vi "teampNight.vi"() -> ()   [LabVIEW 2010]
panel:
  in  "Temp Stop":dbl
  in  "Temp Step":dbl
  in  "Temp Start":dbl
  out "error out":errorcluster
  in  "error in (no error)":errorcluster
  in  "Step":dbl
  in  "Stop":dbl
  in  "Start":dbl
  in  "Path":path
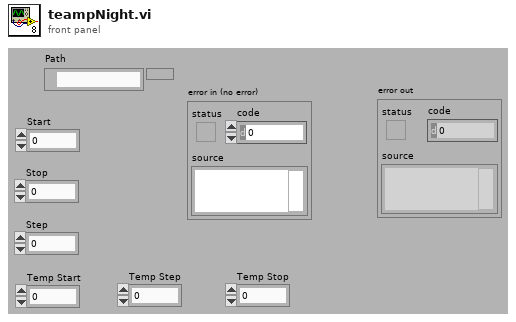
[diagram p1: front panel]
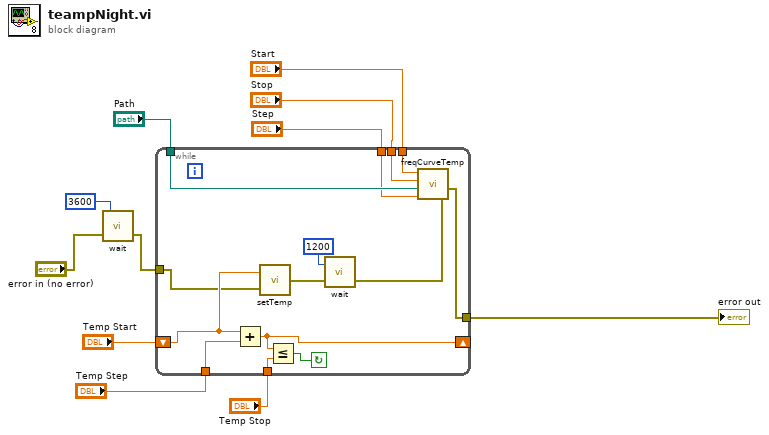
[diagram p0: block diagram]
diagram:
  n1 = call "wait.vi"("error in"="error in (no error)", "Wartezeit in Sek"=3600) -> ("error out"=w1:errorcluster)  [unwired: 1 in]
  n2 = while {
    tunnel: "Path" -> [w25]
    tunnel: w1 -> [w15]
    tunnel: [w24] -> w10
    tunnel: "Start" -> [w22]
    tunnel: "Stop" -> [w21]
    tunnel: "Step" -> [w20]
    shift-right: [w17] -> _
    shift-left: "Temp Start" -> [w16]
    tunnel: "Temp Step" -> [w18]
    tunnel: "Temp Stop" -> [w12]
    stop <- w19 continue-if-true
    n3 = Add(x=w16, y=w18) -> (x+y=w17:dbl)
    n4 = call "setTemp.vi"("error in (no error)"=w15, "Heizspannung"=w16) -> ("error out"=w14:errorcluster)
    n5 = Less Or Equal?(x=w17, y=w12) -> (x <= y?=w19:bool)
    n6 = call "wait.vi"("error in"=w14, "Wartezeit in Sek"=1200) -> ("error out"=w13:errorcluster)  [unwired: 1 in]
    n7 = call "freqCurveTemp.vi"("error in (no error)"=w13, "Step"=w20, "Path"=w25, "End"=w21, "Start"=w22) -> ("error out"=w24:errorcluster)  [unwired: 2 in]
  }
  "error out" <- w10
